vi "Enqueue Targets Update.vi"(2 "error in":errorcluster, 3 "Targets Update":T1={"Valid?"=FALSE, "CapturedAtTimestamp"=0.0, "Targets Message"={"type"="", "message"={"capturedAgoMs"=0, "targets"=[{"x"=0.0, "y"=0.0, "z"=0.0, "theta"=0.0}]}}}, 4 "Targets Queue":refnum<queue>) -> (0 "error out":errorcluster, 1 "Targets Queue":refnum<queue>)   [LabVIEW 2016]
uses:
  Targets Update.ctl
  Targets Message.ctl
  Targets Info.ctl
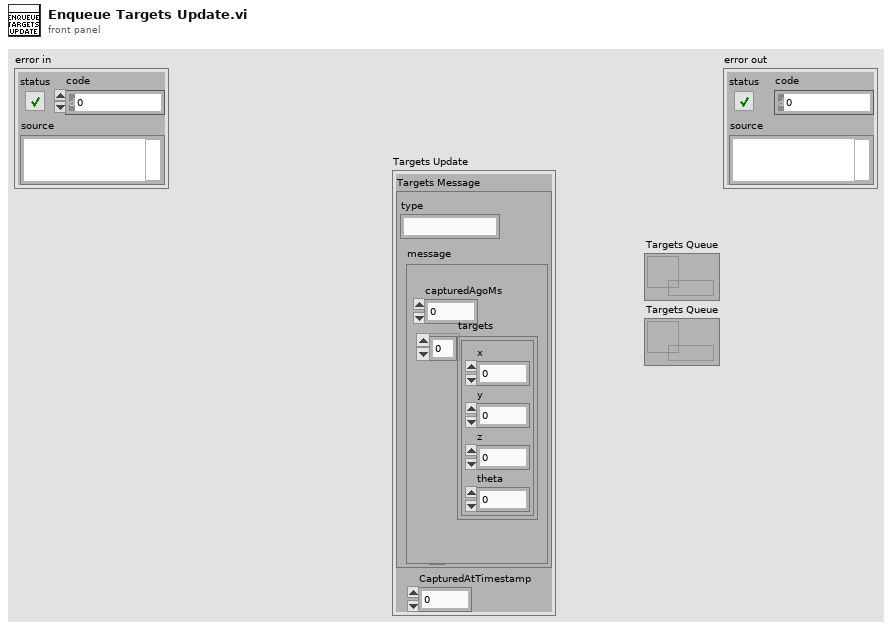
[diagram p1: front panel]
types:
  T1 = typedef "Targets Update.ctl" = cluster{"Valid?":bool, "CapturedAtTimestamp":dbl, "Targets Message":T2}
  T2 = typedef "Targets Message.ctl" = cluster{"type":string, "message":cluster{"capturedAgoMs":i32, "targets":T3[]}}
  T3 = typedef "Targets Info.ctl" = cluster{"x":dbl, "y":dbl, "z":dbl, "theta":dbl}
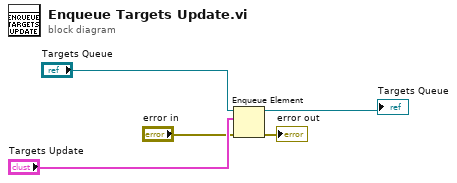
[diagram p0: block diagram]
diagram:
  n1 = Enqueue Element(queue="Targets Queue", element="Targets Update", error in (no error)="error in") -> (queue out=→"Targets Queue":refnum<queue>, error out=→"error out":errorcluster)  [unwired: 1 in, 1 out]
